vi "VFD_Set_Digital.vi"(10 "Control Cluster":T1, 11 "Enable Motor/Pumps\nControl Board":bool) -> ()   [LabVIEW 2021]
uses:
  <vilib>/DAQmx/write.llb/DAQmx Write (Digital 1D Bool NChan 1Samp 1Line).vi
  Human_Labview/global_variables.vi
  <vilib>/DAQmx/create/channels.llb/DAQmx Create Channel (DO-Digital Output).vi
  <vilib>/DAQmx/miscellaneous.llb/DAQmx Fill In Error Info.vi
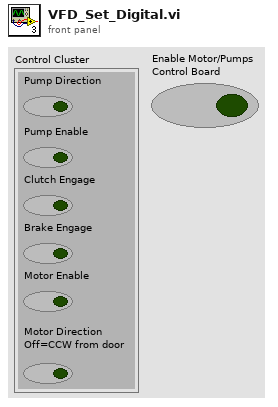
[diagram p1: front panel]
types:
  T1 = cluster{"Pump Direction":bool, "Pump Enable":bool, "Clutch Engage":bool, "Brake Engage":bool, "Motor Enable":bool, "Motor Direction\nOff=CCW from door":bool}
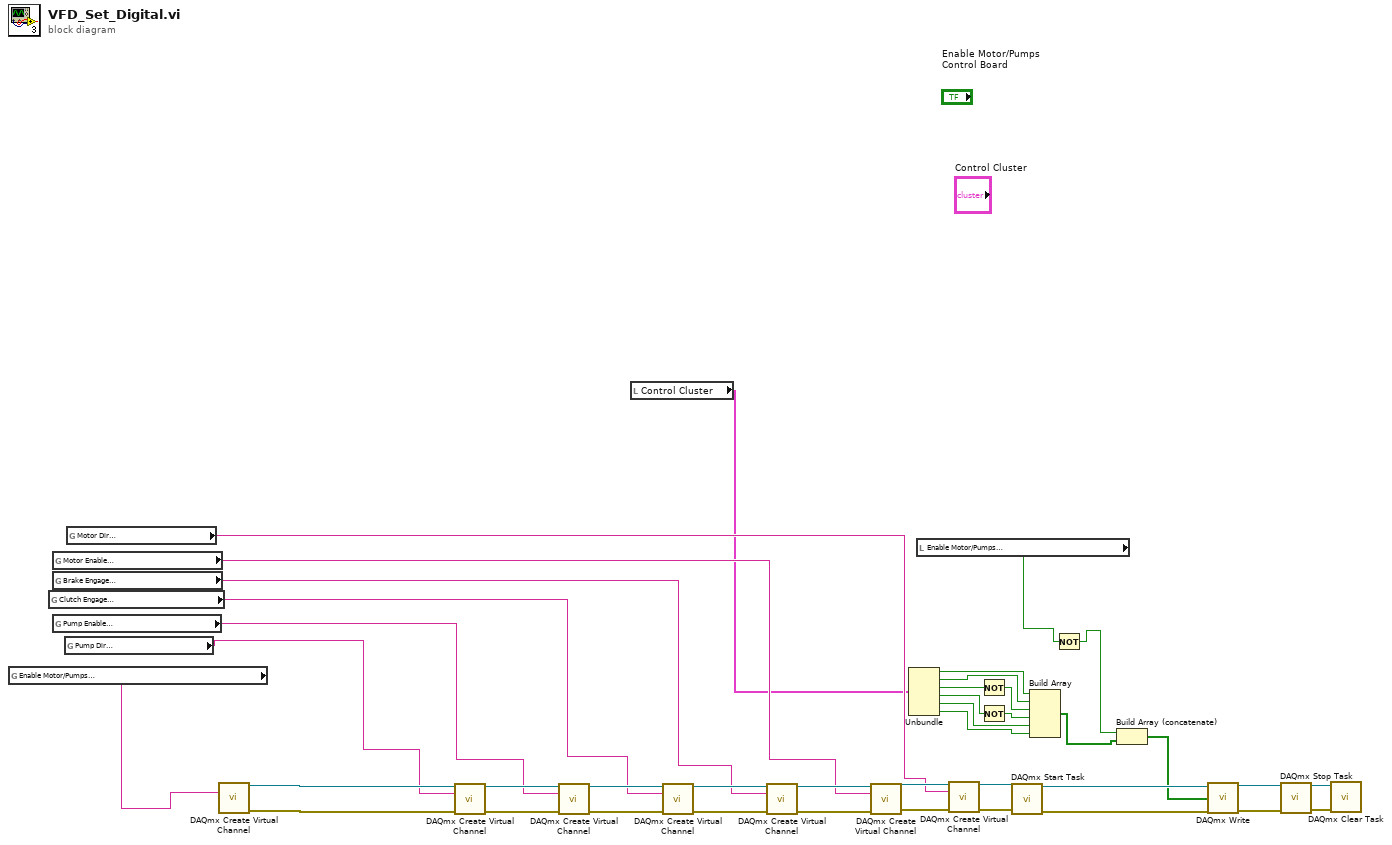
[diagram p0: block diagram]
diagram:
  n1 = global read "global_variables.vi" "Enable Motor/Pumps\nOptical Output Enable"() -> (w4:tag)
  n2 = global read "global_variables.vi" "Clutch Engage\nOptical Out 4"() -> (w12:tag)
  n3 = global read "global_variables.vi" "Motor Enable\nOptical Out 6"() -> (w10:tag)
  n4 = global read "global_variables.vi" "Brake Engage\nOptical Out 5"() -> (w11:tag)
  n5 = global read "global_variables.vi" "Pump Enable\nOptical Out 3"() -> (w13:tag)
  n6 = global read "global_variables.vi" "Pump Dir\nOptical Out 2"() -> (w14:tag)
  n7 = global read "global_variables.vi" "Motor Dir\nOptical Out 7"() -> (w5:tag)
  n8 = call-poly <vilib>:"DAQmx Create Virtual Channel.vi"("lines"=w4) -> ("task out"=w16:refnum<k21>, "error out"=w15:errorcluster)  [unwired: 13 in]
  n9 = call-poly <vilib>:"DAQmx Create Virtual Channel.vi"("task in"=w16, "lines"=w14, "error in"=w15) -> ("task out"=w36:refnum<k21>, "error out"=w32:errorcluster)  [unwired: 11 in]
  n10 = call-poly <vilib>:"DAQmx Create Virtual Channel.vi"("task in"=w36, "lines"=w13, "error in"=w32) -> ("task out"=w35:refnum<k21>, "error out"=w31:errorcluster)  [unwired: 11 in]
  n11 = local read "Control Cluster"() -> (w2:T1)
  n12 = call-poly <vilib>:"DAQmx Create Virtual Channel.vi"("task in"=w35, "lines"=w12, "error in"=w31) -> ("task out"=w34:refnum<k21>, "error out"=w30:errorcluster)  [unwired: 11 in]
  n13 = call-poly <vilib>:"DAQmx Create Virtual Channel.vi"("task in"=w34, "lines"=w11, "error in"=w30) -> ("task out"=w33:refnum<k21>, "error out"=w29:errorcluster)  [unwired: 11 in]
  n14 = call-poly <vilib>:"DAQmx Create Virtual Channel.vi"("task in"=w33, "lines"=w10, "error in"=w29) -> ("task out"=w9:refnum<k21>, "error out"=w8:errorcluster)  [unwired: 11 in]
  n15 = Unbundle(w2) -> ("Pump Direction"=w22:bool, "Pump Enable"=w21:bool, "Clutch Engage"=w28:bool, "Brake Engage"=w27:bool, "Motor Enable"=w25:bool, "Motor Direction\nOff=CCW from door"=w26:bool)
  n16 = local read "Enable Motor/Pumps\nControl Board"() -> (w1:bool)
  n17 = call-poly <vilib>:"DAQmx Create Virtual Channel.vi"("task in"=w9, "lines"=w5, "error in"=w8) -> ("task out"=w7:refnum<k21>, "error out"=w6:errorcluster)  [unwired: 11 in]
  n18 = Not(x=w28) -> (.not. x?=w23:bool)
  n19 = Not(x=w27) -> (.not. x?=w24:bool)
  n20 = call <vilib>:"DAQmx Start Task.vi"("task/channels in"=w7, "error in"=w6) -> ("task out"=w40:refnum<k21>, "error out"=w39:errorcluster)  [unwired: 12 in]
  n21 = Build Array(w22, w21, w23, w24, w25, w26) -> (w20:bool[])
  n22 = Not(x=w1) -> (.not. x?=w3:bool)
  n23 = Build Array (concatenate)(w3, w20) -> (w19:bool[])
  n24 = call-poly <vilib>:"DAQmx Write.vi"("task/channels in"=w40, "data"=w19, "error in"=w39) -> ("task out"=w38:refnum<k21>, "error out"=w37:errorcluster)  [unwired: 10 in, 1 out]
  n25 = call <vilib>:"DAQmx Stop Task.vi"("task/channels in"=w38, "error in"=w37) -> ("task out"=w17:refnum<k21>, "error out"=w18:errorcluster)  [unwired: 12 in]
  n26 = call <vilib>:"DAQmx Clear Task.vi"("task in"=w17, "error in"=w18) -> ()  [unwired: 13 in, 1 out]
